vi "Test Get XML.vi"(11 "Test Case In":refnum<class "Test.Camera.lvclass">) -> (0 "error out":errorcluster, 3 "Test Case Out":refnum<class "Test.Camera.lvclass">)   [LabVIEW 2020, in "Test.Camera.lvclass"]
uses:
  Test.Camera.lvclass
  C:/Program Files (x86)/National Instruments/LabVIEW 2020/vi.lib/Astemes/LUnit/Test Case.lvclass
  g_industrial_cam/Camera/Camera.lvclass/Camera.ctl
  <vilib>/Astemes/LUnit/Test Case.lvclass/Test Case.ctl
  <vilib>/Astemes/LUnit/Append Fail Result.vi
  <vilib>/Astemes/LUnit/Append Pass Result.vi
  <vilib>/Astemes/LUnit/Run In UI.vi
  <vilib>/Utility/error.llb/Clear Errors.vi
  g_industrial_cam/Camera/Check Not Disconnected.vi
  <vilib>/Utility/error.llb/Error Cluster From Error Code.vi
  Test.Camera.lvclass/Test.Camera.ctl
  g_industrial_cam/Camera/Camera.lvclass
  <vilib>/Astemes/LUnit/Test Case.lvclass
panel:
  out "XML":string
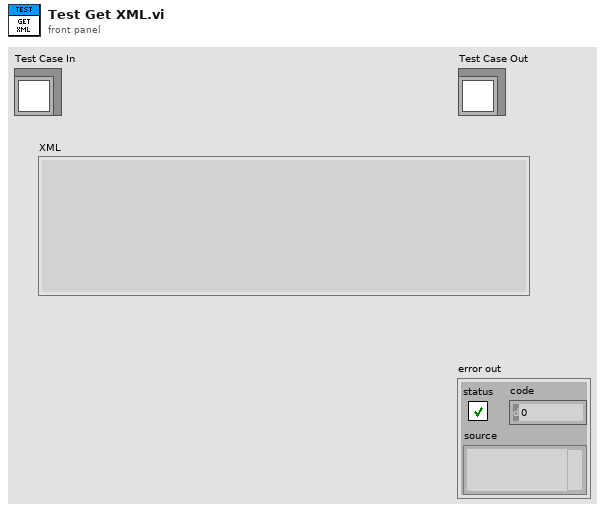
[diagram p1: front panel]
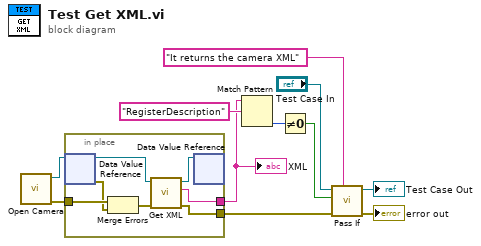
[diagram p0: block diagram]
diagram:
  n1 = call "Open Camera.vi"() -> ("error out"=w2:errorcluster, "Camera"=w3:refnum<data-value>)  [unwired: 10 in]
  n2 = in-place {
    in-place-border: [w18] -> w8
    in-place-border: [w17] -> w1
    in-place-border: w2 -> [w14]
    n3 = in-place-dvr #1(w3) -> (w16:refnum<class "Camera.lvclass">, w13:errorcluster)
    n4 = Merge Errors(w14, w13) -> (w12:errorcluster)
    n5 = call "Get XML.vi"("error in (no error)"=w12, "Camera in"=w16) -> ("error out"=w18:errorcluster, "XML"=w17:string, "Camera"=w15:refnum<class "Camera.lvclass">)  [unwired: 7 in]
    n6 = in-place-dvr #1(w15) -> ()  [unwired: 2 out]
  }
  "XML" <- w1
  n7 = Match Pattern(string=w1, regular expression="RegisterDescription") -> (offset past match=w6:i32)  [unwired: 1 in, 3 out]
  n8 = Not Equal To 0?(x=w6) -> (x != 0?=w5:bool)
  n9 = call <vilib>:"Pass If.vi"("Description"="It returns the camera XML", "error in (no error)"=w8, "Pass?"=w5, "LUnit Test Case In"="Test Case In") -> ("error out"=→"error out":errorcluster, "LUnit Test Case Out"=→"Test Case Out":refnum<class "Test.Camera.lvclass">)  [unwired: 6 in]
